vi "Read Config File.vi"(8 "error in (no error)":errorcluster, 11 "Actor Framework Test in":refnum<class "Actor Framework Test.lvclass">) -> (0 "error out":errorcluster, 3 "Actor Framework Test out":refnum<class "Actor Framework Test.lvclass">)   [LabVIEW 2017, in "Actor Framework Test.lvlib" / "Actor Framework Test.lvclass"]
doc: "Read the configuration file (if it exists) for values that will control this run of the application."
uses:
  Actor Framework Test.lvclass
  Actor Framework Test.lvclass/Actor Framework Test.ctl
  <vilib>/Utility/config.llb/Read Key (I32).vi
  <vilib>/Utility/config.llb/NI_LVConfig.lvlib
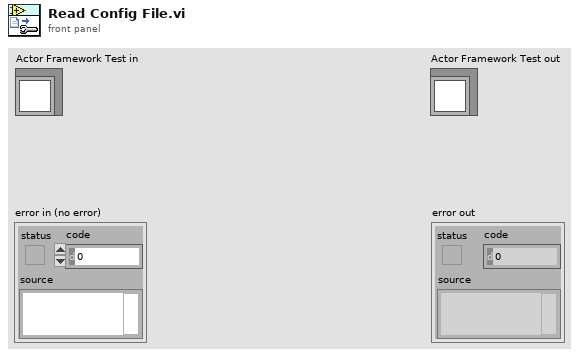
[diagram p1: front panel]
types:
  T1 = typedef "NI_LVConfig.lvlib/Config Data RefNum.ctl" = refnum<k1>
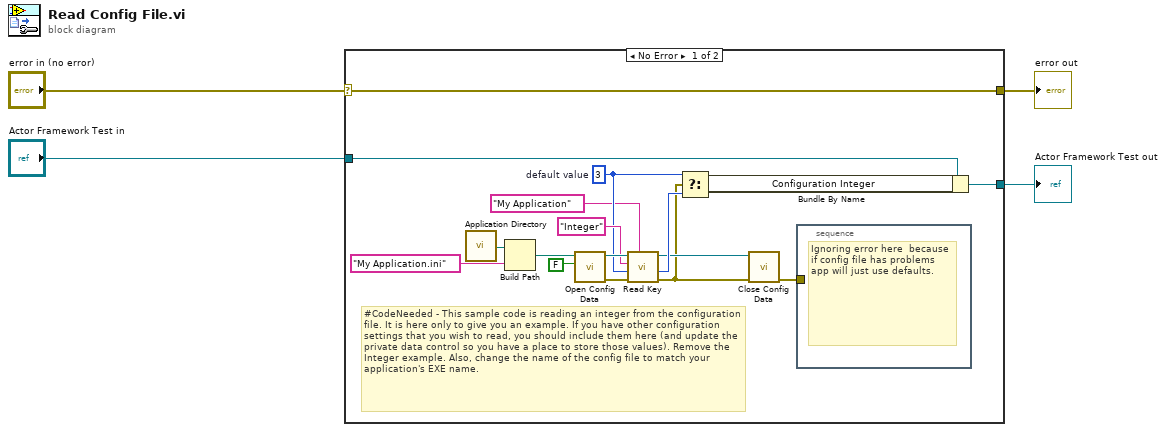
[diagram p0: block diagram]
diagram:
  n1 = case shown="No Error" "error in (no error)" {
    selector: "error in (no error)" -> [w6 w23]
    tunnel: [w6 w23] -> w3
    tunnel: [w10 w22] -> w1
    tunnel: "Actor Framework Test in" -> [w11 w22]
    frame No Error {
      w14 = 3  # default value
      # "#CodeNeeded - This sample code is reading an integer from the configuration file. It is here only to give you an example. If you have other configuration settings that you wish to read, you should include them here (and update the private data control so you have a place to store those values). Remove the Integer example. Also, change the name of the config file to match your application's EXE name."
      n2 = call <vilib>:"Application Directory.vi"() -> ("Application Directory"=w21:path)
      n3 = Build Path(base path=w21, name or relative path="My Application.ini") -> (appended path=w19:path)
      n4 = call <vilib>:"Open Config Data.vi"("create file if necessary (T)"=FALSE, "configuration file path"=w19) -> ("error out"=w17:errorcluster, "refnum"=w16:T1)  [unwired: 7 in, 1 out]
      n5 = call-poly <vilib>:"Read Key.vi"("section"="My Application", "error in (no error)"=w17, "default value"=w14, "key"="Integer", "refnum"=w16) -> ("error out"=w8:errorcluster, "value"=w13:i32, "refnum out"=w9:T1)  [unwired: 3 in, 1 out]
      n6 = Select(t=w14, s=w8, f=w13) -> (s? t:f=w12:i32)
      n7 = Bundle By Name(cluster=w11, "Configuration Integer"=w12) -> (w10:refnum<class "Actor Framework Test.lvclass">)
      n8 = call <vilib>:"Close Config Data.vi"("error in (no error)"=w8, "refnum"=w9) -> ("error out"=w7:errorcluster)  [unwired: 8 in, 1 out]
      n9 = stacked-sequence {
        tunnel: w7 -> [_]
        frame #0 {
          # "Ignoring error here  because if config file has problems app will just use defaults."
        }
      }
    }
    frame Error {
    }
  }
  "error out" <- w3
  "Actor Framework Test out" <- w1
